vi "OAT Cross Point Detection.vi"(2 "pulse width (2)":i32=2, 3 "threshold (0)":dbl format="%.2f", 4 "data in":dbl[](array[numeric]) format="%.2f") -> (1 "edge position":dbl[](array[numeric]) format="%.2f")   [LabVIEW 2017, in "SoundVib_TachProcess.lvlib"]
uses:
  <vilib>/addons/Sound and Vibration/Order Analysis/Tach Process/SoundVib_TachProcess.lvlib
  <vilib>/Analysis/NI_AALPro.lvlib
panel:
  # "Cross Point Detection"
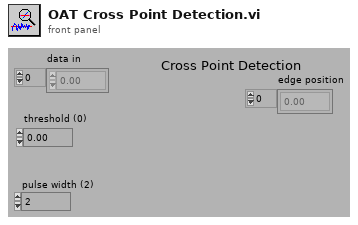
[diagram p1: front panel]
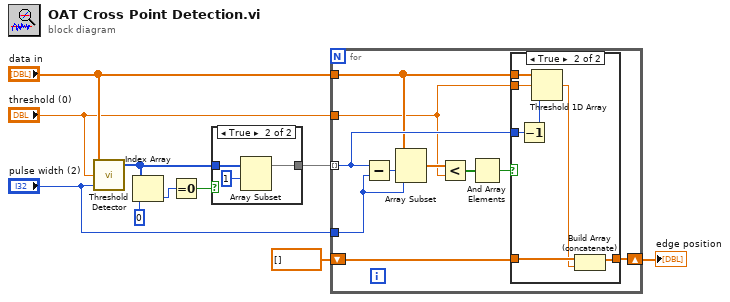
[diagram p0: block diagram]
diagram:
  n1 = call <vilib>:"Threshold Detector.vi"("width"="pulse width (2)", "threshold"="threshold (0)", "X"="data in") -> ("Indices"=w8:i32[])  [unwired: 2 out]
  n2 = Index Array(array=w8, index=0 ("Index")) -> (element=w9:i32)
  n3 = Equal To 0?(x=w9) -> (x = 0?=w7:bool)
  n4 = case shown="True" w7 {
    tunnel: w8 -> [w11 w14]
    tunnel: [w11 w12] -> w6
    frame False {
    }
    frame True {
      n5 = Array Subset(array=w14, index=1 ("Array Index")) -> (w12:i32[])  [unwired: 1 in]
    }
  }
  n6 = for {
    tunnel: w6 -> [w18] mode=indexing
    tunnel: "data in" -> [w16]
    tunnel: "pulse width (2)" -> [w17]
    tunnel: "threshold (0)" -> [w15]
    shift-right: [w21] -> w1
    shift-left: dbl[] [] -> [w20]
    n7 = Subtract(x=w18, y=w17) -> (x-y=w19:i32)
    n8 = Array Subset(array=w16, index=w19, length=w17) -> (w24:dbl[])
    n9 = Less?(x=w24, y=w15) -> (x < y?=w23:bool[])
    n10 = And Array Elements(Boolean array=w23) -> (logical AND=w22:bool)
    n11 = case shown="True" w22 {
      tunnel: w18 -> [_ w30]
      tunnel: [w25 w32] -> w21
      tunnel: w20 -> [w25 w31]
      tunnel: w16 -> [_ w29]
      tunnel: w15 -> [_ w28]
      frame False {
      }
      frame True {
        n12 = Decrement(x=w30) -> (x-1=w27:i32)
        n13 = Threshold 1D Array(1:w27, 2:w28, 3:w29) -> (0:w26:dbl)
        n14 = Build Array (concatenate)(w31, w26) -> (w32:dbl[])
      }
    }
  }
  "edge position" <- w1
